vi "数据解析.vi"(2 "输入":u8[](array[numeric])) -> (0 "ch1":dbl, 1 "ch2":dbl, 3 "ch8":dbl, 4 "ch7":dbl, 5 "ch3":dbl, 6 "ch4":dbl, 7 "ch5":dbl, 8 "ch6":dbl)   [LabVIEW 2018]
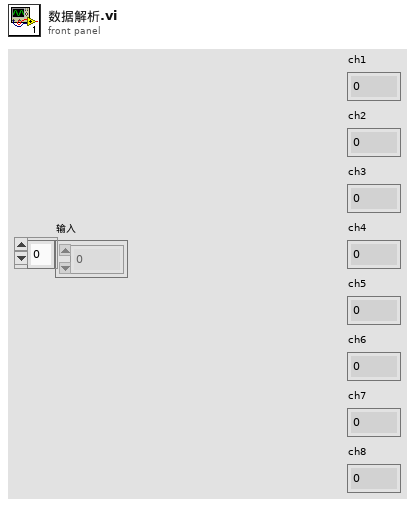
[diagram p1: front panel]
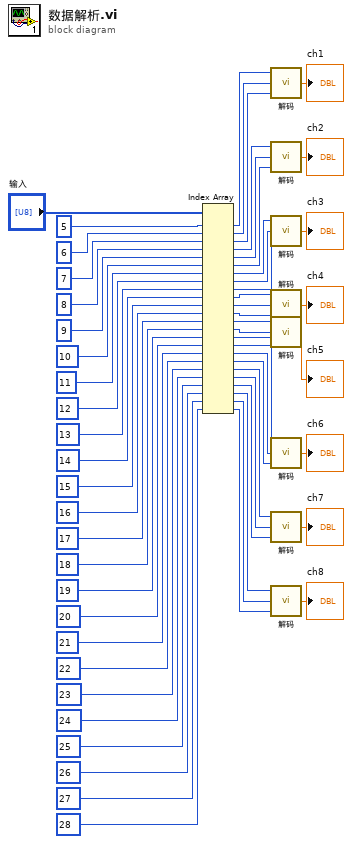
[diagram p0: block diagram]
diagram:
  n1 = Index Array(array="输入", index #1=5 ("索引"), index #2=6 ("索引 2"), index #3=7 ("索引 3"), index #4=8 ("索引"), index #5=9 ("索引"), index #6=10 ("索引"), index #7=11 ("索引"), index #8=12 ("索引"), index #9=13 ("索引"), index #10=14 ("索引"), index #11=15 ("索引"), index #12=16 ("索引"), index #13=17 ("索引"), index #14=18 ("索引"), index #15=19 ("索引"), index #16=20 ("索引"), index #17=21 ("索引"), index #18=22 ("索引"), index #19=23 ("索引"), index #20=24 ("索引"), index #21=25 ("索引"), index #22=26 ("索引"), index #23=27 ("索引"), index #24=28 ("索引")) -> (element #1=w54:u8, element #2=w53:u8, element #3=w52:u8, element #4=w30:u8, element #5=w29:u8, element #6=w28:u8, element #7=w27:u8, element #8=w26:u8, element #9=w25:u8, element #10=w24:u8, element #11=w23:u8, element #12=w22:u8, element #13=w21:u8, element #14=w20:u8, element #15=w19:u8, element #16=w18:u8, element #17=w17:u8, element #18=w16:u8, element #19=w15:u8, element #20=w14:u8, element #21=w13:u8, element #22=w12:u8, element #23=w11:u8, element #24=w10:u8)
  n2 = call "解码.vi"("低8位"=w52, "中8位"=w53, "高8位"=w54) -> ("输出"=→"ch1":dbl)
  n3 = call "解码.vi"("低8位"=w28, "中8位"=w29, "高8位"=w30) -> ("输出"=→"ch2":dbl)
  n4 = call "解码.vi"("低8位"=w25, "中8位"=w26, "高8位"=w27) -> ("输出"=→"ch3":dbl)
  n5 = call "解码.vi"("低8位"=w22, "中8位"=w23, "高8位"=w24) -> ("输出"=→"ch4":dbl)
  n6 = call "解码.vi"("低8位"=w19, "中8位"=w20, "高8位"=w21) -> ("输出"=→"ch5":dbl)
  n7 = call "解码.vi"("低8位"=w16, "中8位"=w17, "高8位"=w18) -> ("输出"=→"ch6":dbl)
  n8 = call "解码.vi"("低8位"=w13, "中8位"=w14, "高8位"=w15) -> ("输出"=→"ch7":dbl)
  n9 = call "解码.vi"("低8位"=w10, "中8位"=w11, "高8位"=w12) -> ("输出"=→"ch8":dbl)
